vi "Web网页服务实验.vi"() -> ()   [LabVIEW 2011]
uses:
  <vilib>/STM32_DriverVI_Interface_F4/Ethernet/IP Type_F4.ctl
  <vilib>/eio/EIO_TerminalDirection.ctl
  <vilib>/STM32_DriverVI_Interface_F4/GPIO_EIO/GPO_EIO_Inner_F4.vi
  <vilib>/eio/EIONode/EIONode.xnode
panel:
  out "Init_Success?":bool
  out "数值":i32
  out "返回字符串":string
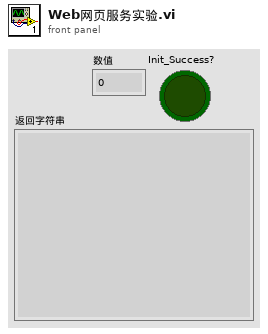
[diagram p1: front panel]
types:
  T1 = typedef "IP Type_F4.ctl" = enum8{"Host IP Address", "Gateway Address", "Subnet Mask Address"}
  T2 = enum8{"P0", "P1", "P2", "P3", "P4", "P5", "P6", "P7", "P8", "P9", "P10", "P11", "P12", "P13", "P14", "P15"}
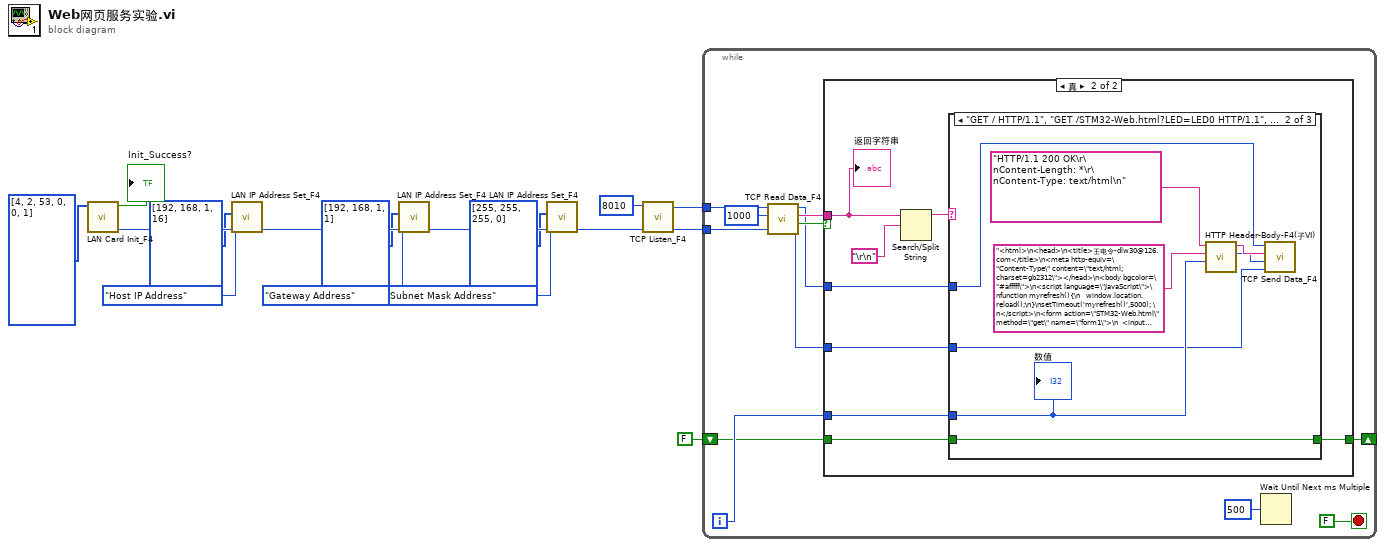
[diagram p0: block diagram]
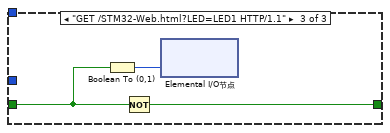
[diagram p4: hidden frame]
diagram:
  n1 = call <vilib>:"LAN Card Init_F4.vi"("MAC_Address（Hex）"=u8[] [4, 2, 53, 0, 0, 1]) -> ("err_out"=w15:u8, "Init_Success?"=→"Init_Success?":bool)  [unwired: 9 in]
  n2 = call <vilib>:"LAN IP Address Set_F4.vi"("err_in"=w15, "IP_Address（Decimal）"=u8[] [192, 168, 1, 16], "IP Address Type"=IP_Type_F4."Host IP Address") -> ("err_out"=w14:u8)  [unwired: 8 in]
  n3 = call <vilib>:"LAN IP Address Set_F4.vi"("err_in"=w14, "IP_Address（Decimal）"=u8[] [192, 168, 1, 1], "IP Address Type"=IP_Type_F4."Gateway Address") -> ("err_out"=w13:u8)  [unwired: 8 in]
  n4 = call <vilib>:"LAN IP Address Set_F4.vi"("err_in"=w13, "IP_Address（Decimal）"=u8[] [255, 255, 255, 0], "IP Address Type"=IP_Type_F4."Subnet Mask Address") -> ("err_out"=w6:u8)  [unwired: 8 in]
  n5 = call <vilib>:"TCP Listen_F4.vi"("err_in"=w6, "Local Port"=u16 8010) -> ("err_out"=w4:u8, "Connect_ID"=w3:u8)  [unwired: 8 in]
  n6 = while {
    tunnel: w4 -> [w28]
    tunnel: w3 -> [w27]
    shift-right: [w17] -> _
    shift-left: FALSE -> [w18]
    i -> [w19]
    stop <- FALSE stop-if-true
    n7 = call <vilib>:"TCP Read Data_F4.vi"("err_in"=w28, "Read_Number（0~1024）"=u16 1000, "Connect_ID"=w27) -> ("err_out"=w22:u8, "Read_Valid?"=w25:bool, "返回字符串"=w24:string, "Connect_ID"=w23:u8)  [unwired: 3 in, 2 out]
    n8 = case shown="真" w25 {
      tunnel: w24 -> [_ w36]
      tunnel: w23 -> [_ w32]
      tunnel: w22 -> [_ w33]
      tunnel: w19 -> [_ w34]
      tunnel: w18 -> [_ w30]
      tunnel: [_ w29] -> w17
      frame False {
      }
      frame True {
        n9 = Search/Split String(string=w36, search string/char (-)="\r\n") -> (substring before match=w35:string)  [unwired: 1 in, 2 out]
        n10 = case shown="\"GET / HTTP/1.1\", \"GET /STM32-Web.html?LED=LED0 HTTP/1.1\", \"POST /STM32-Web.html HTTP/1.1\"" w35 {
          tunnel: w34 -> [_ w42 _]
          tunnel: w33 -> [_ w41 _]
          tunnel: w32 -> [_ w40 _]
          tunnel: [_ w38 w47] -> w29
          tunnel: w30 -> [_ w38 w45]
          frame "假", Default {
          }
          frame "GET / HTTP/1.1", "GET /STM32-Web.html?LED=LED0 HTTP/1.1", "POST /STM32-Web.html HTTP/1.1" {
            n11 = call "HTTP Header-Body-F4(子VI).vi"("循环计数值"=w42, "HTTP Body"="<html>\n<head>\n<title>王电令-dlw30@126.com</title>\n<meta http-equiv=\"Content-Type\" content=\"text/html; charset=gb2312\"></head>\n<body bgcolor=\"#afffff\">\n<script language=\"JavaScript\">\nfunction myrefresh(){\n   window.location.reload();\n}\nsetTimeout('myrefresh()',5000); \n</script>\n<form action=\"STM32-Web.html\" method=\"get\" name=\"form1\">\n  <input type=\"submit\" name=\"LED\" id=\"LED0\" value=\"LED0\">\n  <input type=\"submit\" name=\"LED\" id=\"LED1\" value=\"LED1\">\n  <input type=\"submit\" name=\"LED\" id=\"LED2\" value=\"LED2\">\n  <input type=\"submit\" name=\"LED\" id=\"LED3\" value=\"LED3\">\n  <input type=\"submit\" name=\"LED\" id=\"LED4\" value=\"LED4\">\n  <input type=\"submit\" name=\"LED\" id=\"LED5\" value=\"LED5\"> \n  <input type=\"submit\" name=\"LED\" id=\"PWM-Motor\" value=\"PWM-Motor\">     \n</form>\n<table border=\"0\" width=\"540\">\n<tr>\n<td width=\"14%\">0V</td>\n<td width=\"14%\">0.5V</td>\n<td width=\"14%\">1.5V</td>\n<td width=\"14%\">2.5V</td>\n</tr>\n</table>\n<table bgcolor=\"#FFEEBF\" border=\"5\" cellpadding=\"0\" cellspacing=\"0\" width=\"500\">\n<tr>\n<td>\n<table width=\"temp%\" border=\"0\" cellpadding=\"0\" cellspacing=\"0\">\n<tr><td bgcolor=\"#065fa3\">&nbsp;</td></tr> \n</table>\n</td>\n</tr>\n</table>\n<p>&nbsp;</p>\n</body>\n</html>", "HTTP Header"="HTTP/1.1 200 OK\r\nContent-Length: *\r\nContent-Type: text/html\n") -> ("HTTP Length"=w43:i32, "HTTP File"=w44:string)  [unwired: 7 in]
            n12 = call <vilib>:"TCP Send Data_F4.vi"("err_in"=w41, "Send_Number（0~4096）"=w43, "发送字符串"=w44, "Connect_ID"=w40) -> ()  [unwired: 5 in, 3 out]
            "数值" <- w42
          }
          frame "GET /STM32-Web.html?LED=LED1 HTTP/1.1" {
            n13 = Boolean To (0,1)(Boolean=w45) -> (0, 1=w46:i16)
            n14 = Not(x=w45) -> (.not. x?=w47:bool)
            n15 = xnode "Elemental I/O节点"("LED_1"=w46) -> ()  [unwired: 1 in, 1 out]
          }
        }
        "返回字符串" <- w36
      }
    }
    n16 = Wait Until Next ms Multiple(millisecond multiple=u32 500 ("毫秒倍数")) -> ()  [unwired: 1 out]
  }
